vi "ResMgr-Request SharedDataDVR.vi"(6 "Timeout In ms (5000 ms)":i32=5000, 7 "WatchDogQ":refnum<queue>, 8 "Error In":errorcluster caption="error in (no error)") -> (0 "error out":errorcluster, 3 "DVR":refnum<data-value>)   [LabVIEW 2017, in "Communicable State Machine.lvlib"]
uses:
  Communicable State Machine.lvlib
  CSMQ/_CSMObj-ModeData.ctl
  CSMQ/_CSMObj-Data.ctl
  Typedef/_CSM_MSG_TYPE.ctl
  Priority Queue/Priority Queue.ctl
  Typedef/_Cross CSM State Data.ctl
  Typedef/_Cross CSM State Response.ctl
  Typedef/_CSM_Response Source Message.ctl
  Priority Queue/def-Data(LowPRI-Q).ctl
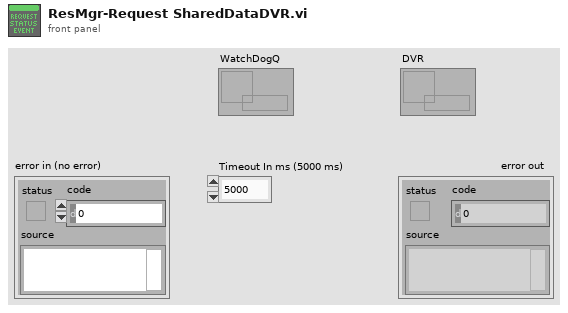
[diagram p1: front panel]
types:
  T1 = typedef "Communicable State Machine.lvlib/_CSMObj-ModeData.ctl" = cluster{"CSMDataDVR":refnum<data-value>[], "PriorityQueues":T2[], "Messages of Chain Nodes":cluster{"Module Name":string, "Allowed Messages":string[]}[], "Chain Message Mapping Map":variant, "SharedRegistryRules":string[]}
  T2 = typedef "Communicable State Machine.lvlib/Priority Queue.ctl" = cluster{"HPriorityQ":refnum<queue>, "LowPriorityQ":refnum<queue>}
  T3 = cluster{"ResType":string, "RespQ":refnum<queue>, "Parameter":string, "WatchDogQ":refnum<queue>}
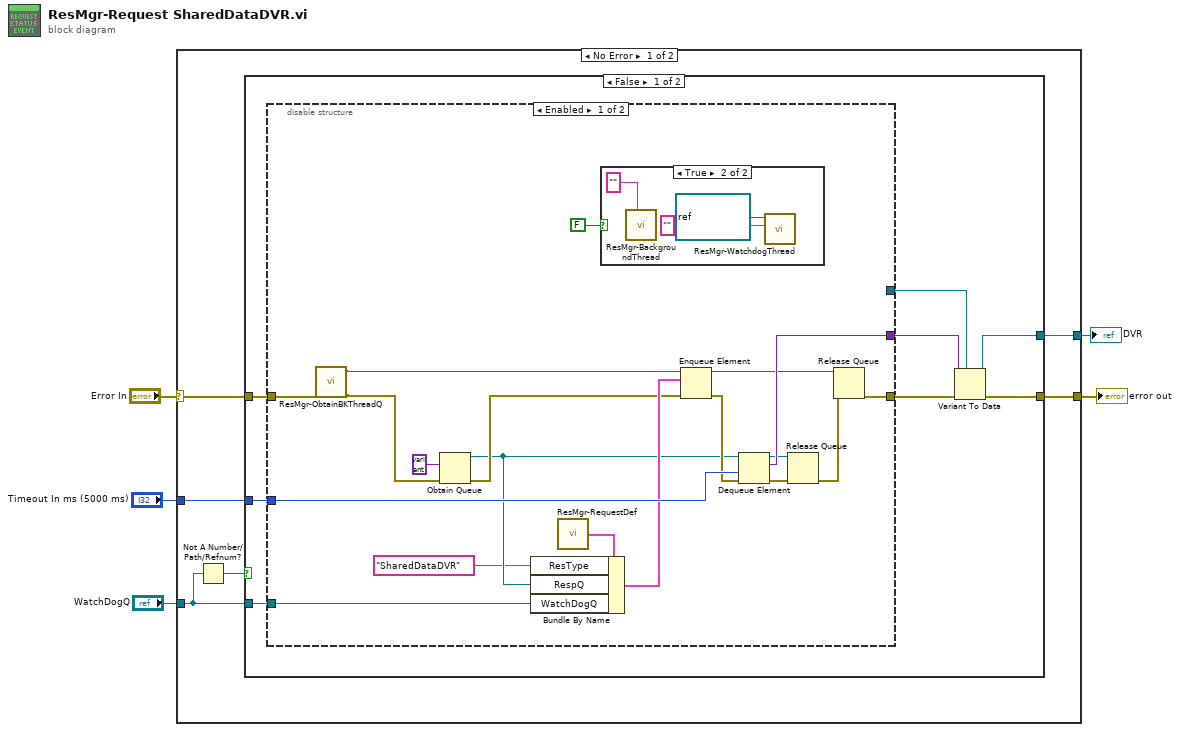
[diagram p0: block diagram]
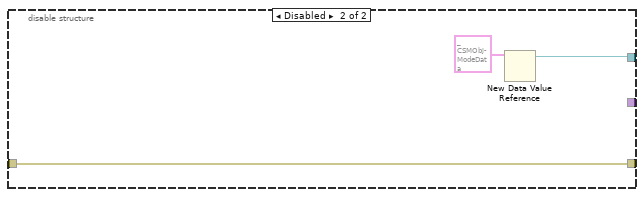
[diagram p3: hidden frame]
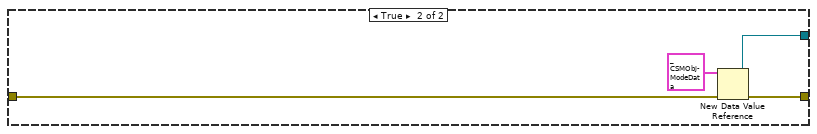
[diagram p4: hidden frame]
diagram:
  n1 = case shown="No Error" "Error In" {
    selector: "Error In" -> [w10 w49]
    tunnel: [w9 w49] -> w5
    tunnel: [w8 _] -> w1
    tunnel: "Timeout In ms (5000 ms)" -> [w11 _]
    tunnel: "WatchDogQ" -> [w7 _]
    frame No Error {
      n2 = Not A Number/Path/Refnum?(number/path/refnum=w7) -> (NaN/Path/Refnum?=w6:bool)
      n3 = case shown="False" w6 {
        tunnel: w11 -> [w18 _]
        tunnel: w10 -> [w17 w47]
        tunnel: w7 -> [w16 _]
        tunnel: [w15 w46] -> w9
        tunnel: [w12 w45] -> w8
        frame False {
          n4 = disable-structure shown="Enabled" {
            disable-tunnel: [w38 w44] -> w19
            disable-tunnel: w18 -> [w37 _]
            disable-tunnel: [w36 _] -> w14
            disable-tunnel: w17 -> [w21 w44]
            disable-tunnel: w16 -> [w25 _]
            disable-tunnel: [_ w42] -> w13
            frame Enabled {
              n5 = call "ResMgr-ObtainBKThreadQ.vi"("error in (no error)"=w21) -> ("error out"=w22:errorcluster, "ObtainBKThreadQ"=w23:refnum<queue>)  [unwired: 9 in]
              n6 = Obtain Queue(element data type=variant, error in (no error)=w22) -> (queue out=w26:refnum<queue>, error out=w34:errorcluster)  [unwired: 3 in, 1 out]
              n7 = call "ResMgr-RequestDef.vi"() -> ("ResMgr-RequestDef.ctl"=w20:T3)  [unwired: 2 in]
              n8 = Bundle By Name(cluster=w20, "ResType"="SharedDataDVR", "RespQ"=w26, "WatchDogQ"=w25) -> (w35:T3)
              n9 = case shown="True" FALSE {
                frame False {
                }
                frame True {
                  n10 = call "ResMgr-BackgroundThread.vi"("Name (Unnamed)"="" ("name (unnamed)")) -> ()  [unwired: 11 in]
                  n11 = call "ResMgr-WatchdogThread.vi"("From Who"="", "WatchDogQ"=refnum<queue> refnum) -> ()  [unwired: 10 in]
                }
              }
              n12 = Enqueue Element(queue=w23, element=w35, error in (no error)=w34) -> (queue out=w30:refnum<queue>, error out=w33:errorcluster)  [unwired: 1 in, 1 out]
              n13 = Dequeue Element(queue=w26, timeout in ms (-1)=w37, error in (no error)=w33) -> (queue out=w31:refnum<queue>, element=w36:variant, error out=w32:errorcluster)  [unwired: 1 out]
              n14 = Release Queue(queue=w31, error in (no error)=w32) -> (error out=w29:errorcluster)  [unwired: 1 in, 2 out]
              n15 = Release Queue(queue=w30, error in (no error)=w29) -> (error out=w38:errorcluster)  [unwired: 1 in, 2 out]
            }
            frame Disabled {
              n16 = New Data Value Reference(data value=T1 {"CSMDataDVR"=[], "PriorityQueues"=[], "Messages of Chain Nodes"=[], "Chain Message Mapping Map"=variant, "SharedRegistryRules"=[]} ("CSMObj-Data")) -> (data value reference=w42:refnum<data-value>)  [unwired: 1 in, 1 out]
            }
          }
          n17 = Variant To Data(error in=w19, type=w13, Variant=w14) -> (data=w12:refnum<data-value>, error out=w15:errorcluster)
        }
        frame True {
          n18 = New Data Value Reference(data value=T1 {"CSMDataDVR"=[], "PriorityQueues"=[], "Messages of Chain Nodes"=[], "Chain Message Mapping Map"=variant, "SharedRegistryRules"=[]} ("CSMObj-Data"), error in=w47) -> (data value reference=w45:refnum<data-value>, error out=w46:errorcluster)
        }
      }
    }
    frame Error {
    }
  }
  "error out" <- w5
  "DVR" <- w1
